vi "has changed dbl first call.vi"(11 "Numeric":dbl) -> (2 "has changed?":bool, 3 "Numeric (dup)":dbl)   [LabVIEW 2021, in "RocketPlot.lvlib"]
uses:
  RocketPlot.lvlib
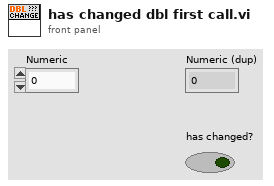
[diagram p1: front panel]
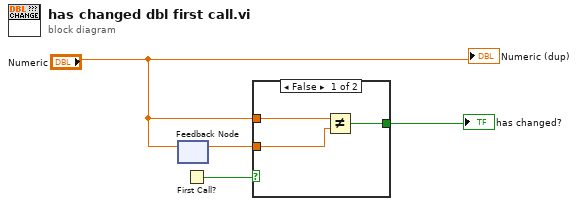
[diagram p0: block diagram]
diagram:
  n1 = feedback-in #1("Numeric") -> ()
  n2 = feedback #1() -> (w4:dbl)  [unwired: 1 in]
  n3 = First Call?() -> (First Call?: T/F=w3:bool)
  n4 = case shown="False" w3 {
    selector: w3 -> [_ w8]
    tunnel: w4 -> [w7 _]
    tunnel: "Numeric" -> [w6 _]
    tunnel: [w5 w8] -> w1
    frame False {
      n5 = Not Equal?(x=w6, y=w7) -> (x != y?=w5:bool)
    }
    frame True {
    }
  }
  "has changed?" <- w1
  "Numeric (dup)" <- "Numeric"
